vi "XYZ Table Stage Module.vi"(6 "Set/Get":T4=enum."Get", 7 "Action":T5, 8 "Error In":errorcluster, 10 "Axis":enum16{"X Axis", "Y Axis", "Z Axis"}(ring), 11 "Table Stages":T3) -> (0 "Error Out":errorcluster, 3 "Table Stages Out":T3)   [LabVIEW 2018]
uses:
  Controls/Motion Translation Module Control.ctl
  General/Controls/Set Get Controls.ctl
  Controls/Translation Stage Cluster.ctl
  General/Controls/Translation Stage Types.ctl
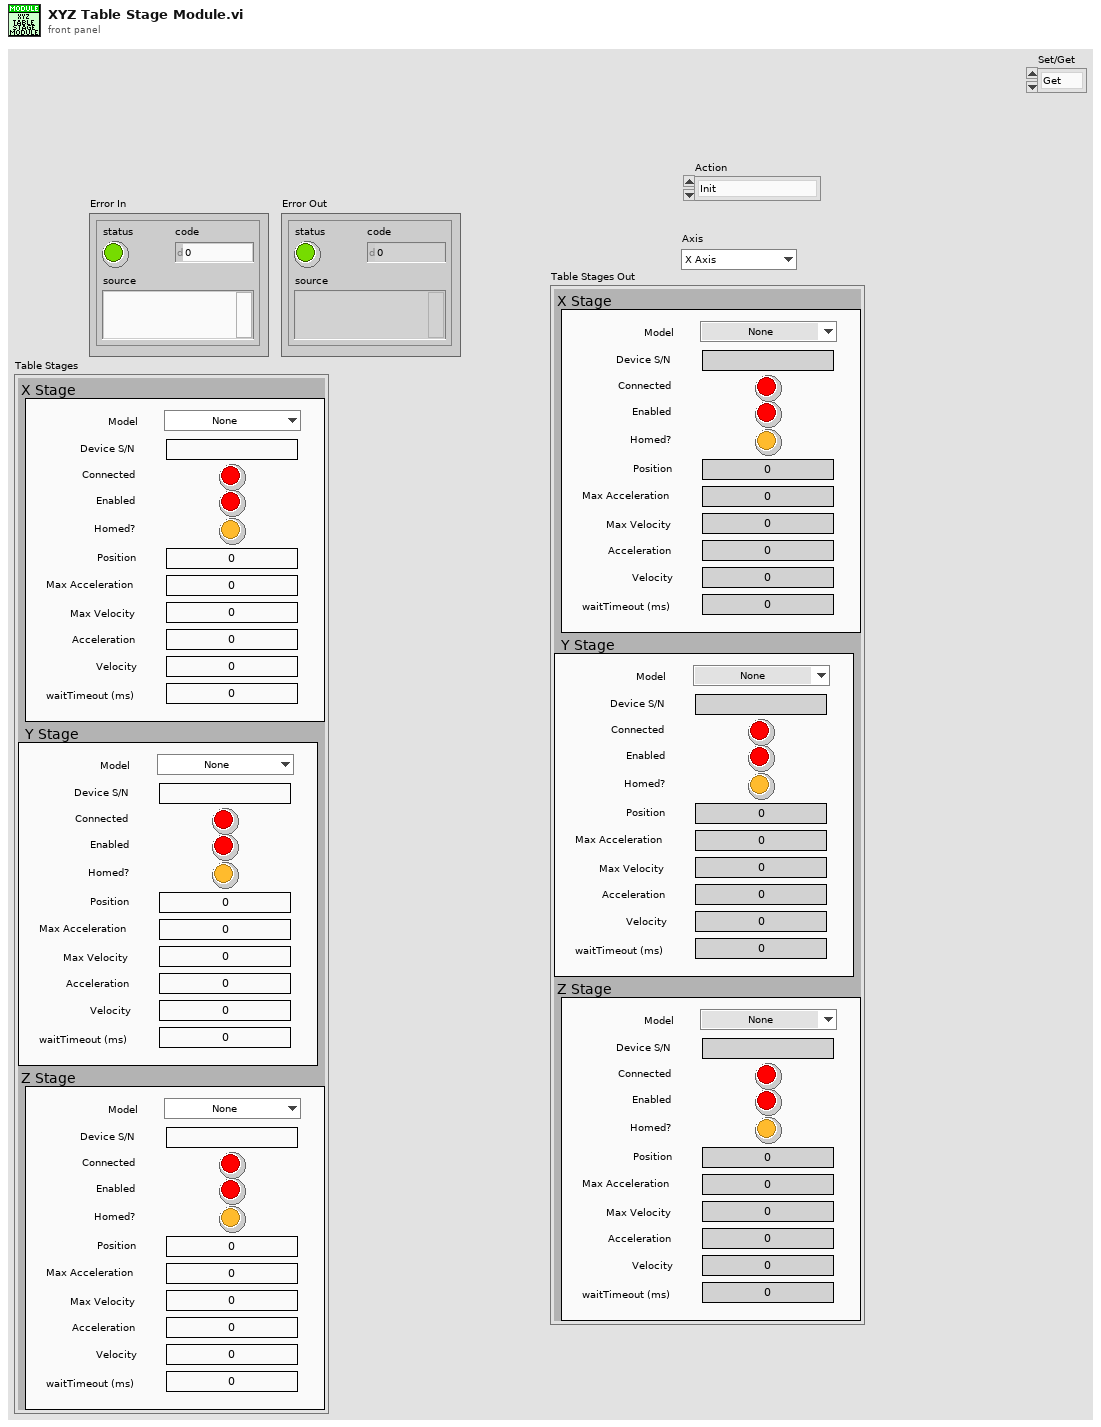
[diagram p1: front panel]
types:
  T1 = typedef "Translation Stage Cluster.ctl" = cluster{"Position":dbl, "Is.Enabled?":bool, "Is.Connected?":bool, "Device SN":string, "AccelerationMaximum":dbl, "VelocityMaximum":dbl, "Acceleration":dbl, "Velocity":dbl, "waitTimeout (ms)":i32, "Model":T2, "Is.Homed?":bool}
  T2 = typedef "Translation Stage Types.ctl" = enum16{"None", "Thorlabs LTS", "Thorlabs MLJ"}
  T3 = cluster{"X Stage":T1, "Y Stage":T1, "Z Stage":T1}
  T4 = typedef "Set Get Controls.ctl" = enum16{"Set", "Get"}
  T5 = typedef "Motion Translation Module Control.ctl" = enum16{"Init", "Home", "Status", "Velocity/Accel", "Position", "Jog", "Stop", "Uninit", "Enable", "Disable"}
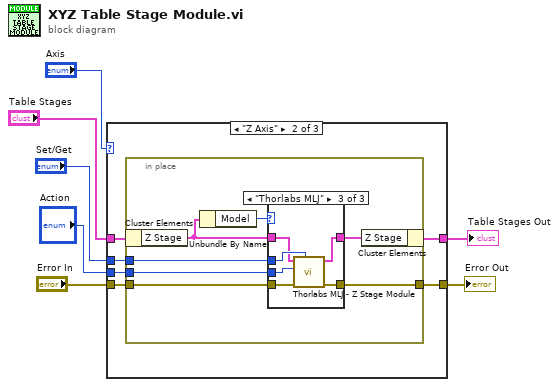
[diagram p0: block diagram]
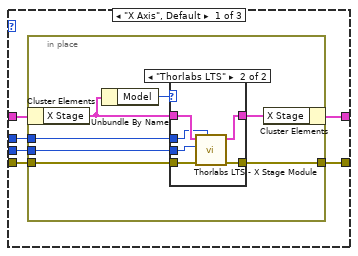
[diagram p2: hidden frame]
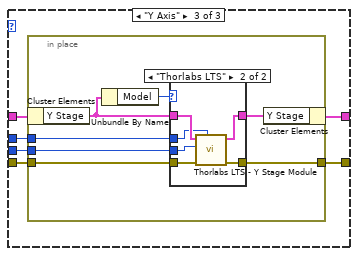
[diagram p6: hidden frame]
diagram:
  n1 = case shown="\"Z Axis\"" "Axis" {
    tunnel: "Set/Get" -> [w10 w32 w54]
    tunnel: "Error In" -> [w13 w34 w57]
    tunnel: "Action" -> [w11 w31 w55]
    tunnel: [w12 w33 w56] -> w5
    tunnel: "Table Stages" -> [w9 w30 w53]
    tunnel: [w8 w29 w52] -> w1
    frame "X Axis", Default {
      n2 = in-place {
        in-place-border: w13 -> [w20]
        in-place-border: [w19] -> w12
        in-place-border: w11 -> [w18]
        in-place-border: w10 -> [w17]
        n3 = in-place-cluster #1(w9) -> ("X Stage"=w15:T1)
        n4 = Unbundle By Name(w15) -> ("Model"=w16:T2)
        n5 = case shown="\"Thorlabs LTS\"" w16 {
          tunnel: w20 -> [w22 w28]
          tunnel: [w22 w27] -> w19
          tunnel: w15 -> [w21 w26]
          tunnel: w18 -> [_ w25]
          tunnel: [w21 w24] -> w14
          tunnel: w17 -> [_ w23]
          frame "None", Default {
          }
          frame "Thorlabs LTS" {
            n6 = call "Thorlabs LTS - X Stage Module.vi"("Set/Get"=w23, "Error In"=w28, "Action"=w25, "Cluster In"=w26) -> ("Error Out"=w27:errorcluster, "Cluster Out"=w24:T1)  [unwired: 6 in]
          }
        }
        n7 = in-place-cluster #1("X Stage"=w14) -> (w8:T3)
      }
    }
    frame "Z Axis" {
      n8 = in-place {
        in-place-border: w34 -> [w41]
        in-place-border: [w40] -> w33
        in-place-border: w32 -> [w39]
        in-place-border: w31 -> [w38]
        n9 = in-place-cluster #2(w30) -> ("Z Stage"=w36:T1)
        n10 = Unbundle By Name(w36) -> ("Model"=w37:T2)
        n11 = case shown="\"Thorlabs MLJ\"" w37 {
          tunnel: w41 -> [w43 w45 w51]
          tunnel: [w43 w45 w50] -> w40
          tunnel: [w42 w44 w49] -> w35
          tunnel: w39 -> [_ _ w48]
          tunnel: w38 -> [_ _ w47]
          tunnel: w36 -> [w42 w44 w46]
          frame "None", Default {
          }
          frame "Thorlabs LTS" {
          }
          frame "Thorlabs MLJ" {
            n12 = call "Thorlabs MLJ - Z Stage Module.vi"("Set/Get"=w48, "Error In"=w51, "Action"=w47, "Cluster In"=w46) -> ("Error Out"=w50:errorcluster, "Cluster Out"=w49:T1)  [unwired: 6 in]
          }
        }
        n13 = in-place-cluster #2("Z Stage"=w35) -> (w29:T3)
      }
    }
    frame "Y Axis" {
      n14 = in-place {
        in-place-border: w57 -> [w64]
        in-place-border: [w63] -> w56
        in-place-border: w55 -> [w62]
        in-place-border: w54 -> [w61]
        n15 = in-place-cluster #3(w53) -> ("Y Stage"=w59:T1)
        n16 = Unbundle By Name(w59) -> ("Model"=w60:T2)
        n17 = case shown="\"Thorlabs LTS\"" w60 {
          tunnel: w64 -> [w66 w72]
          tunnel: [w66 w71] -> w63
          tunnel: [w65 w70] -> w58
          tunnel: w59 -> [w65 w69]
          tunnel: w62 -> [_ w68]
          tunnel: w61 -> [_ w67]
          frame "None", Default {
          }
          frame "Thorlabs LTS" {
            n18 = call "Thorlabs LTS - Y Stage Module.vi"("Set/Get"=w67, "Error In"=w72, "Action"=w68, "Cluster In"=w69) -> ("Error Out"=w71:errorcluster, "Cluster Out"=w70:T1)  [unwired: 6 in]
          }
        }
        n19 = in-place-cluster #3("Y Stage"=w58) -> (w52:T3)
      }
    }
  }
  "Error Out" <- w5
  "Table Stages Out" <- w1
